vi "Read IMU Data.vi"(8 "error in (no error)":errorcluster, 11 "LINX-SenseHat in":refnum<class "LINX-SenseHat.lvclass">) -> (0 "error out":errorcluster, 2 "IMU Data":T1, 3 "LINX-SenseHat out":refnum<class "LINX-SenseHat.lvclass">)   [LabVIEW 2020, in "LINX-SenseHat.lvclass"]
uses:
  LINX-SenseHat.lvclass
  LSM9DS1/LSM9DS1 IMU.lvclass
  LSM9DS1/3 Axis Values.ctl
  IMU Data.ctl
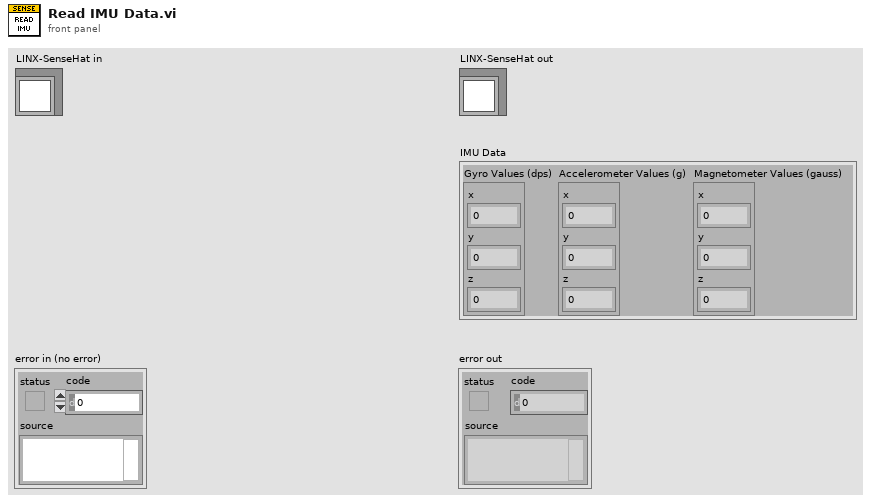
[diagram p1: front panel]
types:
  T1 = typedef "LINX-SenseHat.lvclass/IMU Data.ctl" = cluster{"Gyro Values (dps)":T2, "Accelerometer Values (g)":T2, "Magnetometer Values (gauss)":T2}
  T2 = typedef "LSM9DS1 IMU.lvclass/3 Axis Values.ctl" = cluster{"x":dbl, "y":dbl, "z":dbl}
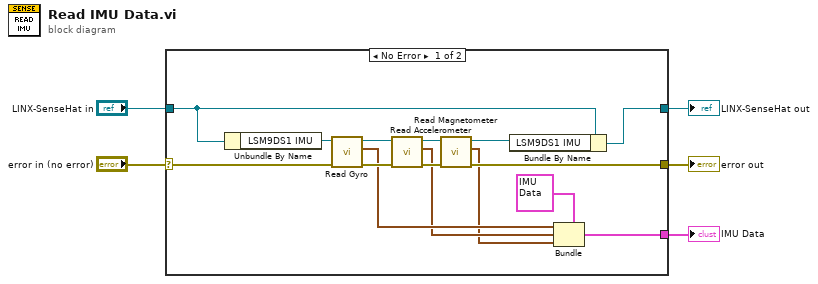
[diagram p0: block diagram]
diagram:
  n1 = case shown="No Error" "error in (no error)" {
    selector: "error in (no error)" -> [w11 w22]
    tunnel: [w12 w22] -> w4
    tunnel: [w19 w21] -> w2
    tunnel: "LINX-SenseHat in" -> [w20 w21]
    tunnel: [w7 _] -> w1
    frame No Error {
      n2 = Unbundle By Name(w20) -> ("LSM9DS1 IMU"=w13:refnum<class "LSM9DS1 IMU.lvclass">)
      n3 = call "Read Gyro.vi"("error in (no error)"=w11, "LSM9DS1 IMU in"=w13) -> ("error out"=w17:errorcluster, "Gyro Values (dps)"=w10:T2, "LSM9DS1 IMU out"=w18:refnum<class "LSM9DS1 IMU.lvclass">)  [unwired: 7 in]
      n4 = call "Read Accelerometer.vi"("error in (no error)"=w17, "LSM9DS1 IMU in"=w18) -> ("error out"=w15:errorcluster, "Accelerometer Values (g)"=w9:T2, "LSM9DS1 IMU out"=w16:refnum<class "LSM9DS1 IMU.lvclass">)  [unwired: 7 in]
      n5 = call "Read Magnetometer.vi"("error in (no error)"=w15, "LSM9DS1 IMU in"=w16) -> ("error out"=w12:errorcluster, "Magnetometer Values (gauss)"=w8:T2, "LSM9DS1 IMU out"=w14:refnum<class "LSM9DS1 IMU.lvclass">)  [unwired: 7 in]
      n6 = Bundle By Name(cluster=w20, "LSM9DS1 IMU"=w14) -> (w19:refnum<class "LINX-SenseHat.lvclass">)
      n7 = Bundle(cluster=T1 {"Gyro Values (dps)"={"x"=0.0, "y"=0.0, "z"=0.0}, "Accelerometer Values (g)"={"x"=0.0, "y"=0.0, "z"=0.0}, "Magnetometer Values (gauss)"={"x"=0.0, "y"=0.0, "z"=0.0}} ("IMU Data"), "Gyro Values (dps)"=w10, "Accelerometer Values (g)"=w9, "Magnetometer Values (gauss)"=w8) -> (w7:T1)
    }
    frame Error {
    }
  }
  "error out" <- w4
  "LINX-SenseHat out" <- w2
  "IMU Data" <- w1
